vi "Set XYZ Voltage.vi"(6 "Set Z Voltage(V)":dbl, 8 "error in (no error)":errorcluster, 9 "Set Y Voltage(V)":dbl, 10 "Set x Voltage(V)":dbl, 11 "hdl in":i32) -> (0 "error out":errorcluster, 3 "hdl":i32)   [LabVIEW 2011, in "Thorlabs_MDT69xB.lvlib"]
doc: "Set xyz voltage, only valid for MDT 693B three channel controller."
uses:
  <instrlib>/Thorlabs_MDT69xB/Thorlabs_MDT69xB.lvlib
  <instrlib>/Thorlabs_MDT69xB/Data/MDT_COMMAND_LIB_win32.dll
  <instrlib>/Thorlabs_MDT69xB/Data/MDT_COMMAND_LIB_x64.dll
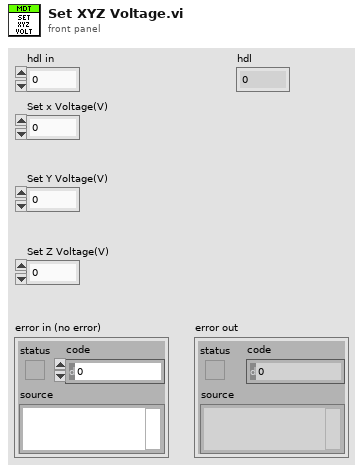
[diagram p1: front panel]
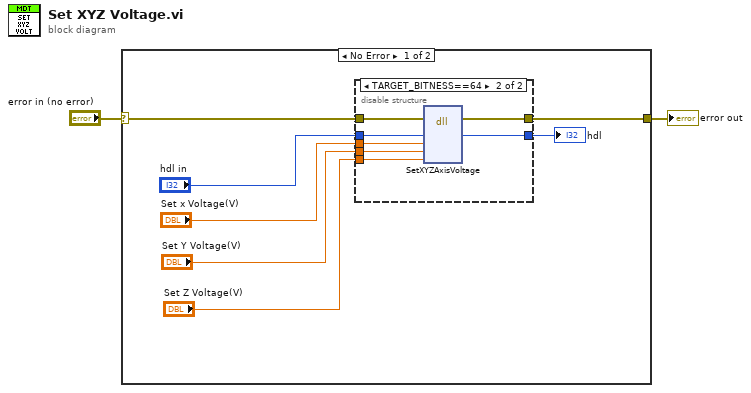
[diagram p0: block diagram]
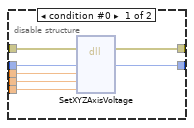
[diagram p2: hidden frame]
diagram:
  n1 = case shown="No Error" "error in (no error)" {
    selector: "error in (no error)" -> [w9 w24]
    tunnel: [w6 w24] -> w1
    frame No Error {
      n2 = disable-structure shown="TARGET_BITNESS==64" {
        disable-tunnel: w9 -> [w16 w23]
        disable-tunnel: "hdl in" -> [w15 w22]
        disable-tunnel: "Set x Voltage(V)" -> [w14 w21]
        disable-tunnel: [w13 w20] -> w6
        disable-tunnel: [w12 w19] -> w5
        disable-tunnel: "Set Y Voltage(V)" -> [w11 w18]
        disable-tunnel: "Set Z Voltage(V)" -> [w10 w17]
        frame condition #0 {
          n3 = dll-call lib="E:/Program Files (x86)/National Instruments/LabVIEW 2011/instr.lib/Thorlabs_MDT69xB/Data/MDT_COMMAND_LIB_win32.dll" fn="SetXYZAxisVoltage"(error in=w16, "hdl"=w15, "X voltage"=w14, "Y voltage"=w11, "Z voltage"=w10) -> (error out=w13:errorcluster, "hdl"=w12:i32)  [unwired: 6 in, 1 out]
        }
        frame condition #1 (active) {
          n4 = dll-call lib="C:/Program Files/National Instruments/LabVIEW 2011/instr.lib/Thorlabs_MDT69xB/Data/MDT_COMMAND_LIB_x64.dll" fn="SetXYZAxisVoltage"(error in=w23, "hdl"=w22, "X voltage"=w21, "Y voltage"=w18, "Z voltage"=w17) -> (error out=w20:errorcluster, "hdl"=w19:i32)  [unwired: 6 in, 1 out]
        }
      }
      "hdl" <- w5
    }
    frame Error {
    }
  }
  "error out" <- w1
